vi "FineContrast.vi"(0 "LightField Automation":refnum<class "LightField Automation.lvclass">, 1 "PZC200 Instrument Channel":string="GPIB/0:4,0", 3 "PZC Error":errorcluster, 4 "Acq Time (ms) 2":dbl=500.0 caption="Acq Time :" min=0.0 max=360000.0 step=50.0, 5 "Acq Mode":T1=enum."Spectrum" caption="Mode :", 6 "CCD ROI":T2(ring), 7 "LightField Automation error":errorcluster, 8 "Shutter Device Reference":refnum<vi>, 9 "PZC Position Readout (usteps) 2":refnum<vi>, 10 "LinTFine Start":dbl, 11 "LinTFine End":dbl, 12 "Shutter Controls":refnum<vi>, 13 "Scan Spectrum Progess Bar 2":refnum<vi>, 14 "Stop Contrast 2":refnum<vi>, 15 "Pause Contrast 2":refnum<vi>, 16 "Contrast 1D Spectrum 2":refnum<vi>, 17 "LinTFine Step":dbl, 18 "Accumulations":dbl, 19 "Contrast Oscillations 2":refnum<vi>) -> (20 "LightField Automation out":refnum<class "LightField Automation.lvclass">, 21 "PZC200 Instrument Channel 2":string, 24 "PZC Error 2":errorcluster, 25 "PZA Positions":i32[](array[numeric]), 26 "Spectra vs PZA":i32[][](array[numeric]), 27 "LightField Automation error  out":errorcluster)   [LabVIEW 2019]
uses:
  D:/Users/manip-thz/Documents/Controle_Manip_2020/Thorlabs.MotionControl.KCube.SolenoidCLI.dll
  Thorlabs.MotionControl.KCube.SolenoidCLI.dll
  Light Field/lightfield-automation-labview/LightField Automation.lvclass
  TypeDefs/AcqMode.ctl
panel:
  out "WavelengthCalibration":dbl[](array[numeric])
  out "x+y":dbl
  out "Contrast values":i32[](array[numeric])
  out "Contrast 1D Spectrum":cluster{dbl[], dbl[]}(graph) caption="64.0°"
  out "Contrast Oscillations":cluster{dbl[], dbl[]}(graph)
  in  "Pause Contrast":bool
  in  "Stop Contrast":bool
  out "PZC Position Readout (usteps)":dbl caption="Readout (usteps)" min=-8.0 max=392.0
  out "Scan Spectrum Progess Bar":u8(slide) scale=0.0..100.0
  out "KCube Shutter Device Reference":refnum<k24>
  out "Shutter Ctrls":u16(ring)
  # "ms"
types:
  T1 = typedef "AcqMode.ctl" = enum16{"Image", "Spectrum", "APD 1", "APD 2", "APD 1+2"}
  T2 = enum16{"Custom ROI", "Full sensor", "Binned full sensor"}
  T3 = enum16{"Contrast", "Spectre", "Polarisation", "XY Intensity Map"}
  T4 = enum16{"Image", "Spectrum", "APD 1", "APD 2", "APD 1+2"}
  T5 = cluster{"Image":dbl[][][], "Frame Size":cluster{"F":i32, "Y":i32, "X":i32}}[]
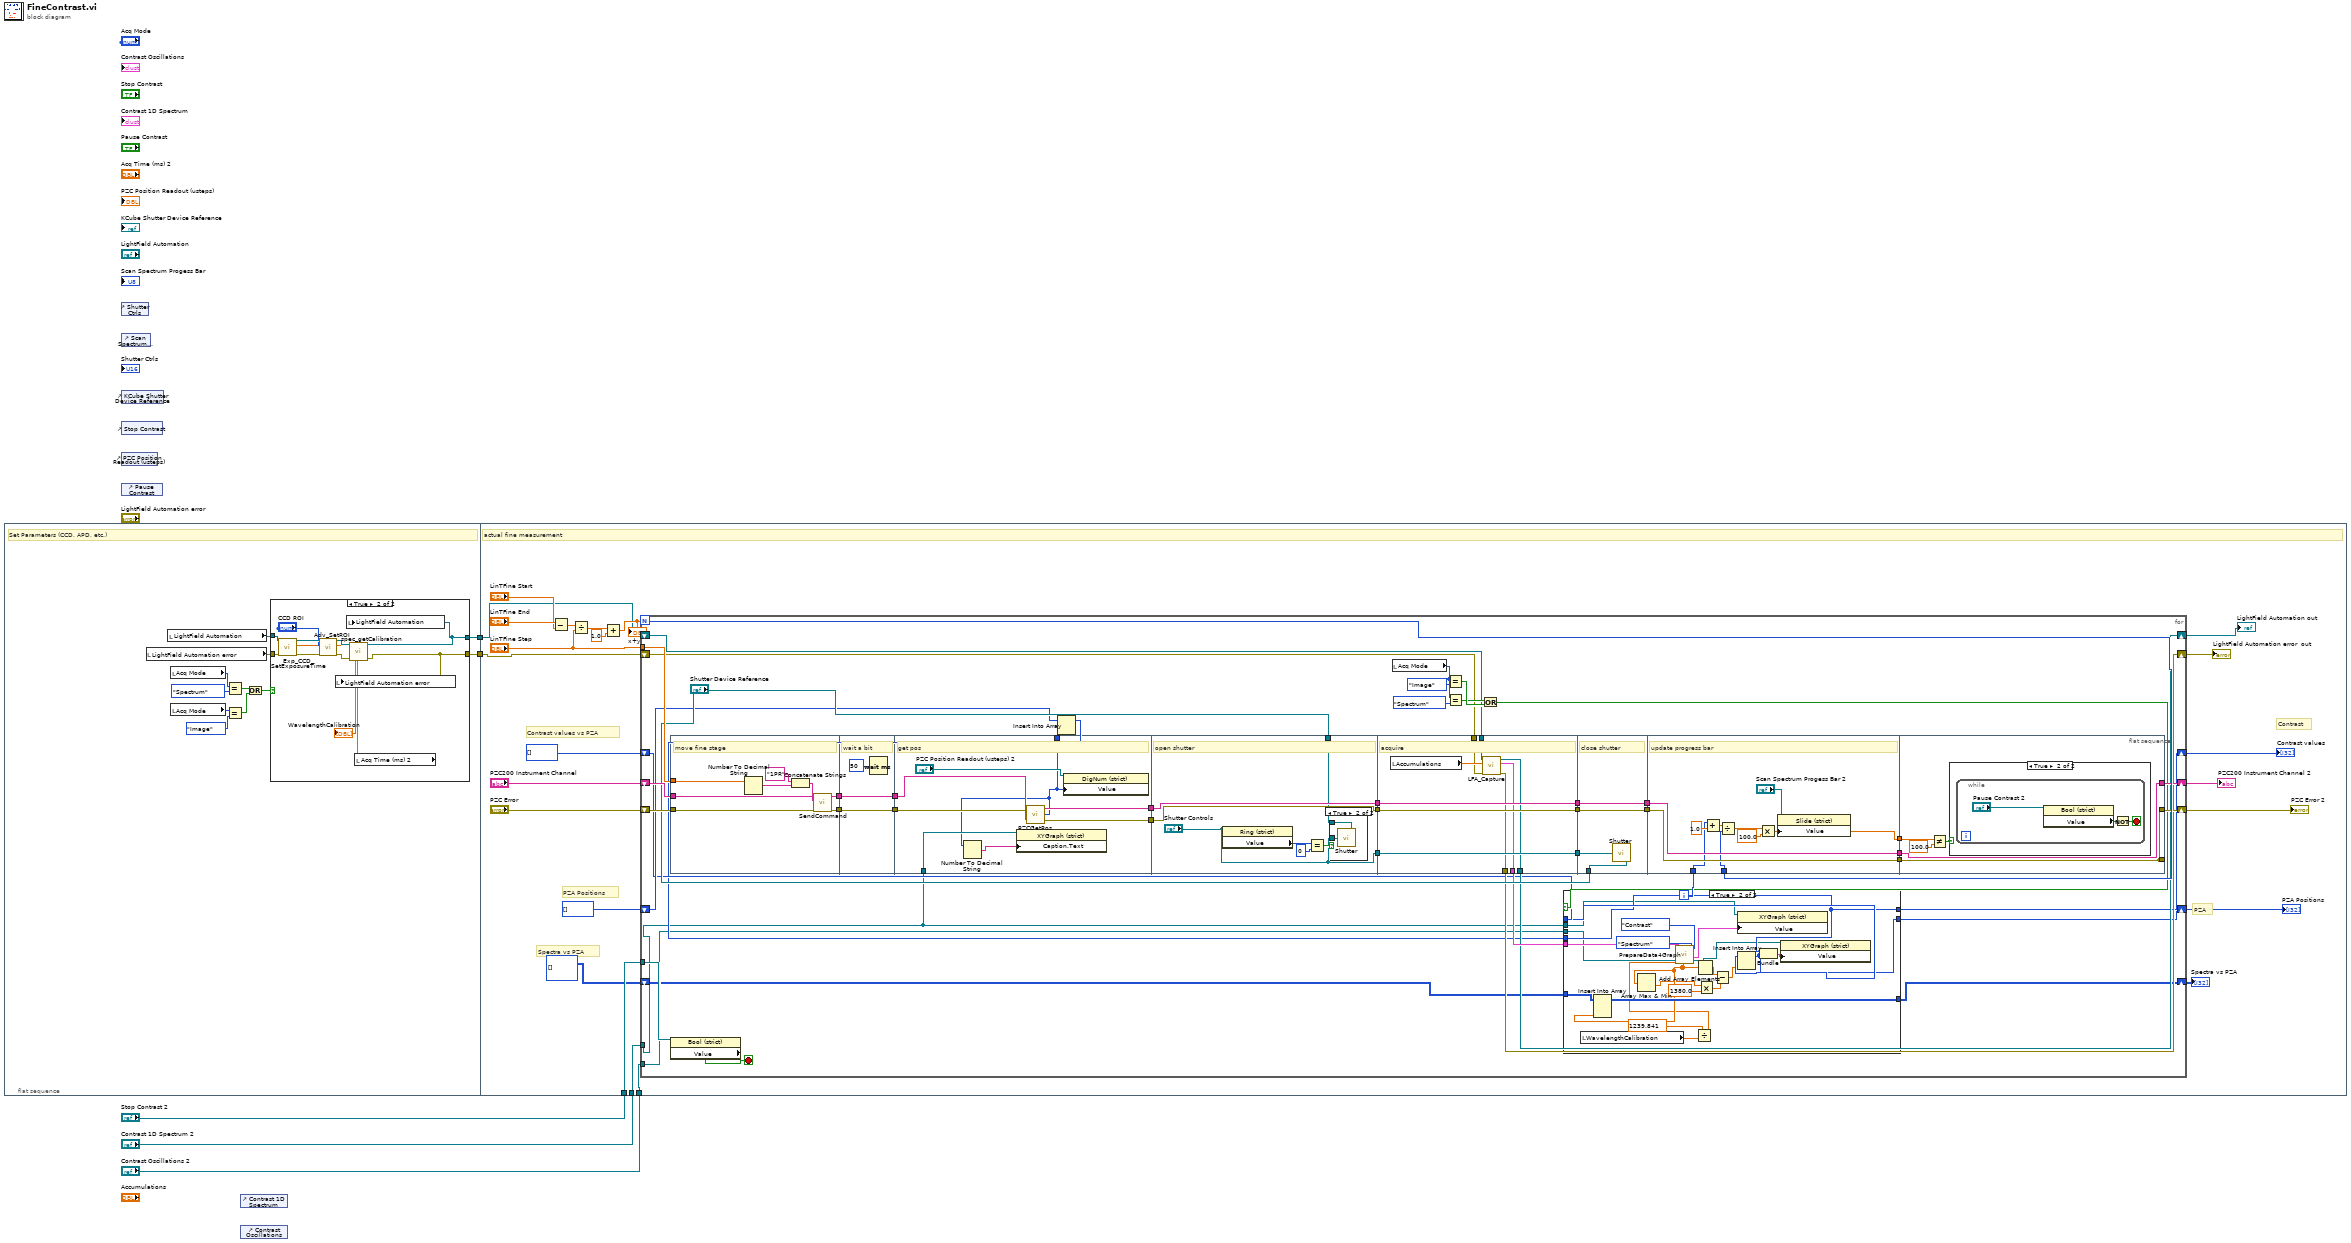
[diagram p0: block diagram]
diagram:
  n1 = flat-sequence {
    tunnel: [w9] -> w5
    tunnel: [w8] -> w4
    tunnel: w5 -> [w42]
    tunnel: w4 -> [w41]
    tunnel: "Stop Contrast 2" -> [w34]
    tunnel: "Contrast 1D Spectrum 2" -> [w33]
    tunnel: "Contrast Oscillations 2" -> [w32]
    frame #0 {
      # "Set Parameters (CCD, APD, etc.)"
      n2 = local read "LightField Automation error"() -> (w7:errorcluster)
      n3 = local read "LightField Automation"() -> (w6:refnum<class "LightField Automation.lvclass">)
      n4 = local read "Acq Mode"() -> (w16:T1)
      n5 = local read "Acq Mode"() -> (w12:T1)
      n6 = Equal?(x=w16, y=AcqMode."Spectrum" ("Acq Mode")) -> (x = y?=w14:bool)
      n7 = Equal?(x=w12, y=AcqMode."Image" ("Acq Mode")) -> (x = y?=w11:bool)
      n8 = Or(x=w14, y=w11) -> (x .or. y?=w10:bool)
      n9 = case shown="True" w10 {
        tunnel: [w18 w22] -> w9
        tunnel: [w17 w21] -> w8
        tunnel: w7 -> [w17 w26]
        tunnel: w6 -> [w18 w25]
        frame False {
        }
        frame True {
          n10 = local read "Acq Time (ms) 2"() -> (w19:dbl)
          n11 = call "Exp_CCD_SetExposureTime.vi"("error in (no error)"=w26, "Exposure Time (s)"=w19, "LightField Automation in"=w25) -> ("error out"=w28:errorcluster, "LightField Automation out"=w29:refnum<class "LightField Automation.lvclass">)  [unwired: 7 in]
          n12 = call "Adv_SetROI.vi"("error in (no error)"=w28, "ROI"="CCD ROI", "LightField Automation in"=w29) -> ("error out"=w23:errorcluster, "LightField Automation out"=w24:refnum<class "LightField Automation.lvclass">)  [unwired: 7 in]
          n13 = call "spec_getCalibration.vi"("error in (no error)"=w23, "LightField Automation in"=w24) -> ("error out"=w21:errorcluster, "ColumnCalibration"=→"WavelengthCalibration":dbl[], "LightField Automation out"=w22:refnum<class "LightField Automation.lvclass">)  [unwired: 7 in]
          n14 = local write "LightField Automation error"(w21) -> ()
          n15 = local write "LightField Automation"(w22) -> ()
        }
      }
    }
    frame #1 {
      # "Spectra vs PZA"
      # "Contrast"
      # "PZA"
      # "Contrast values vs PZA"
      # "PZA Positions"
      # "actual fine measurement"
      n16 = Subtract(x="LinTFine End", y="LinTFine Start") -> (x-y=w51:dbl)
      n17 = Divide(x=w51, y="LinTFine Step") -> (x/y=w50:dbl)
      n18 = Add(x=w50, y=1.0) -> (x+y=w48:dbl)
      "x+y" <- w48
      n19 = for {
        N: w48 -> [w85]
        tunnel: "LinTFine Step" -> [w101]
        shift-right: [w80] -> w44
        shift-left: "PZC200 Instrument Channel" -> [w99]
        shift-right: [w79] -> w43
        shift-left: "PZC Error" -> [w100]
        shift-right: [w66] -> w40
        shift-left: w42 -> [w68]
        shift-right: [w65] -> w39
        shift-left: w41 -> [w67]
        shift-right: [w60] -> w35
        shift-left: i32[] [] -> [w63]
        shift-right: [w59] -> w36
        shift-left: i32[] [] -> [w62]
        tunnel: w34 -> [w58]
        tunnel: w33 -> [w54]
        tunnel: w32 -> [w57]
        shift-right: [w55] -> w30
        shift-left: i32[][] [] -> [w56]
        i -> [w86]
        stop <- w81 stop-if-true
        n20 = flat-sequence {
          tunnel: w101 -> [w133]
          tunnel: [w129] -> w98
          tunnel: [w128] -> w96
          tunnel: w100 -> [w127]
          tunnel: w99 -> [w126]
          tunnel: w98 -> [w136]
          tunnel: [w136] -> w97
          tunnel: w96 -> [w135]
          tunnel: [w135] -> w95
          tunnel: w97 -> [w144]
          tunnel: w95 -> [w143]
          tunnel: [w142] -> w94
          tunnel: [w141] -> w93
          tunnel: [w137] -> w64
          tunnel: w54 -> [w139]
          tunnel: w94 -> [w151]
          tunnel: w93 -> [w150]
          tunnel: "Shutter Device Reference" -> [w146]
          tunnel: [w151] -> w92
          tunnel: [w150] -> w91
          tunnel: ["Shutter Controls"] -> w77
          tunnel: w92 -> [w162]
          tunnel: w91 -> [w161]
          tunnel: [w162] -> w90
          tunnel: [w161] -> w89
          tunnel: [w159] -> w78
          tunnel: w77 -> [w159]
          tunnel: [w158] -> w75
          tunnel: w68 -> [w157]
          tunnel: w67 -> [w156]
          tunnel: [w155] -> w66
          tunnel: [w154] -> w65
          tunnel: w90 -> [w166]
          tunnel: w89 -> [w165]
          tunnel: [w166] -> w88
          tunnel: [w165] -> w87
          tunnel: w78 -> [w164]
          tunnel: "Shutter Device Reference" -> [w163]
          tunnel: w88 -> [w176]
          tunnel: w87 -> [w175]
          tunnel: w86 -> [w169]
          tunnel: w85 -> [w168]
          tunnel: [w176] -> w84
          tunnel: [w175] -> w83
          tunnel: [w167] -> w82
          tunnel: [w177] -> _
          tunnel: [w181] -> w80
          tunnel: w84 -> [w181]
          tunnel: w83 -> [w177]
          tunnel: w82 -> [w179]
          tunnel: [w177] -> w79
          frame #0 {
            # "move fine stage"
            n21 = Number To Decimal String(number=w133) -> (decimal integer string=w131:string)  [unwired: 1 in]
            n22 = Concatenate Strings("1PR", w131) -> (w130:string)
            n23 = call "SendCommand.vi"("error in"=w127, "Command"=w130, "Instrument Channel"=w126) -> ("error out"=w128:errorcluster, "Instrument Channel out"=w129:string)  [unwired: 7 in]
          }
          frame #1 {
            # "wait a bit"
            n24 = Wait (ms)(milliseconds to wait=u32 50) -> ()  [unwired: 1 out]
          }
          frame #2 {
            # "get pos"
            n25 = call "PZCGetPos.vi"("error in"=w143, "Instrument Channel"=w144) -> ("Instrument Channel Out"=w142:string, "Position"=w137:i32, "error out"=w141:errorcluster)
            n26 = Number To Decimal String(number=w137) -> (decimal integer string=w138:string)  [unwired: 1 in]
            n27 = property class="XYGraph (strict)"(reference=w139, "Caption.Text"=w138) -> ()  [unwired: 1 in, 2 out]
            n28 = property class="DigNum (strict)"(reference="PZC Position Readout (usteps) 2", "Value"=w137) -> ()  [unwired: 1 in, 2 out]
          }
          frame #3 {
            # "open shutter"
            n29 = property class="Ring (strict)"(reference="Shutter Controls") -> ("Value"=w147:u16)  [unwired: 1 in, 2 out]
            n30 = Equal?(x=w147, y=u16 0) -> (x = y?=w148:bool)
            n31 = case shown="True" w148 {
              tunnel: "Shutter Controls" -> [_ w153]
              tunnel: w146 -> [_ w152]
              frame False {
              }
              frame True {
                n32 = call "Shutter.vi"("KCube Shutter Device Reference 2"=w152, "Shutter Ctrls 2"=w153) -> ()
              }
            }
          }
          frame #4 {
            # "acquire"
            n33 = local read "Accumulations"() -> (w160:dbl)
            n34 = call "LFA_Capture.vi"("error in (no error)"=w156, "Frames"=w160, "LightField Automation in"=w157) -> ("error out"=w154:errorcluster, "Data"=w158:T5, "LightField Automation out"=w155:refnum<class "LightField Automation.lvclass">)  [unwired: 6 in]
          }
          frame #5 {
            # "close shutter"
            n35 = call "Shutter.vi"("KCube Shutter Device Reference 2"=w163, "Shutter Ctrls 2"=w164) -> ()
          }
          frame #6 {
            # "update progress bar"
            n36 = Add(x=w169, y=1.0) -> (x+y=w173:dbl)
            n37 = Divide(x=w173, y=w168) -> (x/y=w172:dbl)
            n38 = Multiply(x=w172, y=100.0) -> (x*y=w167:dbl)
            n39 = property class="Slide (strict)"(reference="Scan Spectrum Progess Bar 2", "Value"=w167) -> ()  [unwired: 1 in, 2 out]
          }
          frame #7 {
            n40 = Not Equal?(x=w179, y=100.0) -> (x != y?=w178:bool)
            n41 = case shown="True" w178 {
              frame False {
              }
              frame True {
                n42 = while {
                  stop <- w183 stop-if-true
                  n43 = property class="Bool (strict)"(reference="Pause Contrast 2") -> ("Value"=w184:bool)  [unwired: 1 in, 2 out]
                  n44 = Not(x=w184) -> (.not. x?=w183:bool)
                }
              }
            }
          }
        }
        n45 = property class="Bool (strict)"(reference=w58) -> ("Value"=w81:bool)  [unwired: 1 in, 2 out]
        n46 = Insert Into Array(array=w63, new element=w64) -> (w61:i32[])  [unwired: 1 in]
        n47 = local read "Acq Mode"() -> (w74:T1)
        n48 = Equal?(x=w74, y=AcqMode."Image" ("Acq Mode")) -> (x = y?=w71:bool)
        n49 = Equal?(x=w74, y=AcqMode."Spectrum" ("Acq Mode")) -> (x = y?=w70:bool)
        n50 = Or(x=w70, y=w71) -> (x .or. y?=w69:bool)
        n51 = case shown="True" w69 {
          tunnel: w75 -> [_ w125]
          tunnel: w62 -> [w103 w124]
          tunnel: w61 -> [w104 w122]
          tunnel: [w104 w122] -> w60
          tunnel: [w103 w121] -> w59
          tunnel: w54 -> [_ w120]
          tunnel: w57 -> [_ w119]
          tunnel: w56 -> [w102 w115]
          tunnel: [w102 w114] -> w55
          frame False {
          }
          frame True {
            n52 = local read "WavelengthCalibration"() -> (w107:dbl[])
            n53 = Divide(x=1239.841, y=w107) -> (x/y=w105:dbl[])
            n54 = call "PrepareData4Graph.vi"("Wavelength nm"=w105, "DataLF"=w125, "AcqMode"=T4."Spectrum", "Data type"=T3."Contrast") -> ("Spectrum"=w116:cluster{"Array 2":dbl[], "Array":dbl[]}, "PLInt out"=w110:dbl[])  [unwired: 2 in, 2 out]
            n55 = Insert Into Array(array=w115, new element=w110) -> (w114:i32[][])  [unwired: 2 in]
            n56 = Array Max & Min(array=w110) -> (min value=w109:dbl)  [unwired: 3 out]
            n57 = Add Array Elements(numeric array=w110) -> (sum=w113:dbl)
            n58 = Multiply(x=w109, y=1380.0) -> (x*y=w108:dbl)
            n59 = Subtract(x=w113, y=w108) -> (x-y=w112:dbl)
            n60 = property class="XYGraph (strict)"(reference=w120, "Value"=w116) -> ()  [unwired: 1 in, 2 out]
            n61 = Insert Into Array(array=w124, new element=w112) -> (w121:i32[])  [unwired: 1 in]
            n62 = Bundle(w122, w121) -> (w123:cluster{i32[], i32[]})  [unwired: 1 in]
            n63 = property class="XYGraph (strict)"(reference=w119, "Value"=w123) -> ()  [unwired: 1 in, 2 out]
          }
        }
      }
      "LightField Automation out" <- w40
      "LightField Automation error  out" <- w39
      "Contrast values" <- w36
      "PZA Positions" <- w35
      "PZC Error 2" <- w43
      "PZC200 Instrument Channel 2" <- w44
      "Spectra vs PZA" <- w30
    }
  }
  n64 = control-ref of="Shutter Ctrls"() -> ()  [unwired: 1 out]
  n65 = control-ref of="Scan Spectrum Progess Bar"() -> ()  [unwired: 1 out]
  n66 = control-ref of="KCube Shutter Device Reference"() -> ()  [unwired: 1 out]
  n67 = control-ref of="Stop Contrast"() -> ()  [unwired: 1 out]
  n68 = control-ref of="PZC Position Readout (usteps)"() -> ()  [unwired: 1 out]
  n69 = control-ref of="Pause Contrast"() -> ()  [unwired: 1 out]
  n70 = control-ref of="Contrast 1D Spectrum"() -> ()  [unwired: 1 out]
  n71 = control-ref of="Contrast Oscillations"() -> ()  [unwired: 1 out]
